vi "List Required Keys.vi"(10 "Runtime Implementation":T1) -> (1 "Initial Values":string[](array[string]), 2 "Requested Keys":string[](array[string]))   [LabVIEW 2015, in "E2E Tag Exchange configuration.lvclass"]
uses:
  module/configuration/E2E Tag Exchange configuration.lvclass
  module/configuration/Runtime Implementation.ctl
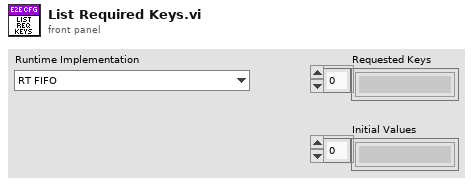
[diagram p1: front panel]
types:
  T1 = typedef "E2E Tag Exchange configuration.lvclass/Runtime Implementation.ctl" = enum16{"RT FIFO", "UDP"}
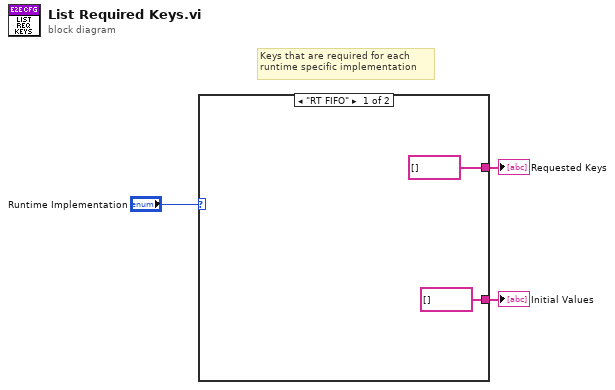
[diagram p0: block diagram]
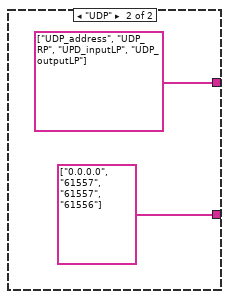
[diagram p2: hidden frame]
diagram:
  # "Keys that are required for each\nruntime specific implementation"
  n1 = case shown="\"RT FIFO\"" "Runtime Implementation" {
    tunnel: [string[] [] string[] ["UDP_address", "UDP_RP", "UPD_inputLP", "UDP_outputLP"]] -> w2
    tunnel: [string[] [] string[] ["0.0.0.0", "61557", "61557", "61556"]] -> w1
    frame "RT FIFO" {
    }
    frame "UDP" {
    }
  }
  "Requested Keys" <- w2
  "Initial Values" <- w1
